vi "Link Splitter References.vi"(8 "error in (no error)":errorcluster, 11 "Main in":refnum<class "Main.lvclass">) -> (0 "error out":errorcluster, 3 "Main out":refnum<class "Main.lvclass">)   [LabVIEW 2023, in "Main.lvlib" / "Main.lvclass"]
uses:
  Library/Main.lvclass
  Library/Main.lvclass/Main.ctl
  builds/Framework/Engine.lvlibp/Engine/Accessors/Read VI Ref.vi
  builds/Main/Docking.lvlibp/Docking/Write Splitter Refnum.vi
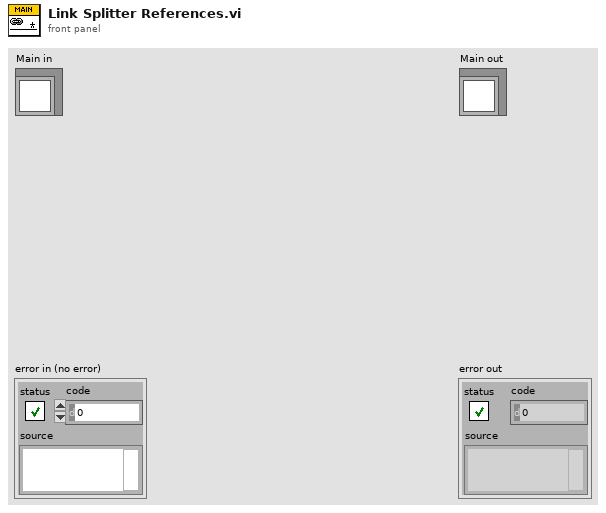
[diagram p1: front panel]
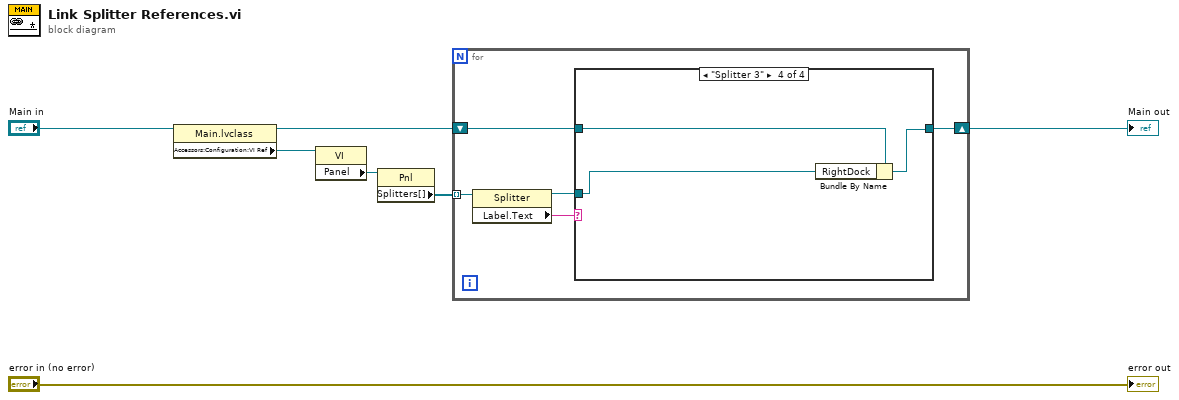
[diagram p0: block diagram]
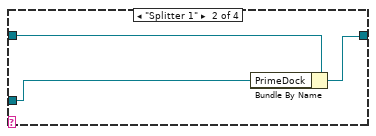
[diagram p3: hidden frame]
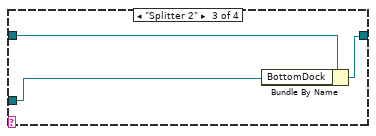
[diagram p4: hidden frame]
diagram:
  n1 = property class="Main.lvclass"(reference="Main in") -> (reference out=w6:refnum<class "Main.lvclass">, "Accessors:Configuration:VI Ref"=w4:refnum<vi>)  [unwired: 1 in, 1 out]
  n2 = property class="VI"(reference=w4) -> ("Panel"=w5:refnum<vi>)  [unwired: 1 in, 2 out]
  n3 = property class="Pnl"(reference=w5) -> ("Splitters[]"=w7:refnum<vi>[])  [unwired: 1 in, 2 out]
  n4 = for {
    shift-right: [w9] -> w2
    shift-left: w6 -> [w10]
    tunnel: w7 -> [w12] mode=indexing
    n5 = property class="Splitter"(reference=w12) -> (reference out=w8:refnum<vi>, "Label.Text"=w11:string)  [unwired: 1 in, 1 out]
    n6 = case shown="\"Splitter 3\"" w11 {
      tunnel: w10 -> [w13 w16 w19 w22]
      tunnel: [w13 w15 w18 w21] -> w9
      tunnel: w8 -> [_ w14 w17 w20]
      frame "False", Default {
      }
      frame "Splitter 1" {
        n7 = Bundle By Name(cluster=w16, "PrimeDock"=w14) -> (w15:refnum<class "Main.lvclass">)
      }
      frame "Splitter 2" {
        n8 = Bundle By Name(cluster=w19, "BottomDock"=w17) -> (w18:refnum<class "Main.lvclass">)
      }
      frame "Splitter 3" {
        n9 = Bundle By Name(cluster=w22, "RightDock"=w20) -> (w21:refnum<class "Main.lvclass">)
      }
    }
  }
  "Main out" <- w2
  "error out" <- "error in (no error)"
